vi "SetGreenLevel.vi"(0 "error in":errorcluster, 2 "Green Light \nLevel":sgl, 3 "node":string) -> (1 "error out":errorcluster)   [LabVIEW 2015]
doc: "Sets the green light on Baxter's head to a given level"
uses:
  ROS/Code/Console/Servers/ServerSubs/TopicDef.ctl
  ROS/Code/SubVIs/_ROSDirection.ctl
  ROS/MessageBuilding/std_msgs/subs/float32Scalar.vi
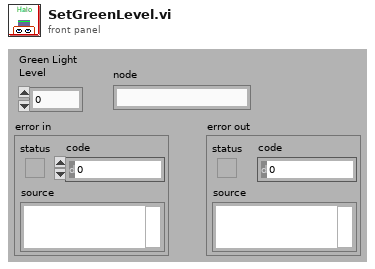
[diagram p1: front panel]
types:
  T1 = typedef "TopicDef.ctl" = cluster{"Topic":string, "Type":string, "Action":T2, "Update (ms)":u16, "queue size":u16}
  T2 = typedef "_ROSDirection.ctl" = enum16{"Node", "Publisher", "Subscriber", "ServiceClient", "ServiceProvider"}
  T3 = typedef "_ROSControl.ctl" = cluster{"topic port":u16, "Node":string, "topic":string, "type":string, "node port":u16, "error ":errorcluster, "Direction":T2, "Update (ms)":u16, "FIFO size":u16}
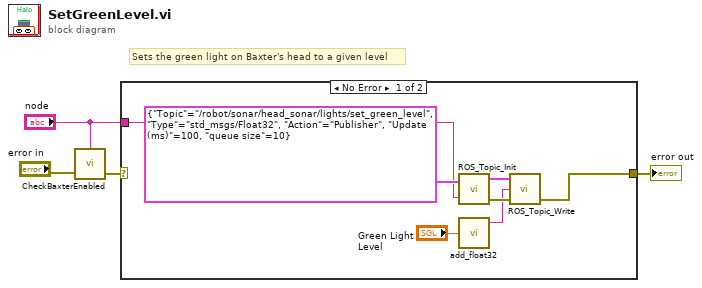
[diagram p0: block diagram]
diagram:
  # "Sets the green light on Baxter's head to a given level"
  n1 = call "CheckBaxterEnabled.vi"("error in"="error in", "node"="node") -> ("error out"=w2:errorcluster)  [unwired: 2 in]
  n2 = case shown="No Error" w2 {
    selector: w2 -> [_ w12]
    tunnel: [w5 w12] -> w4
    tunnel: "node" -> [w8 _]
    frame No Error {
      n3 = call "ROS_Topic_Init.vi"("Definitions"=T1 {"Topic"="/robot/sonar/head_sonar/lights/set_green_level", "Type"="std_msgs/Float32", "Action"=enum."Publisher", "Update (ms)"=100, "queue size"=10}, "node"=w8) -> ("ROS out"=w11:T3, "error out"=w7:errorcluster)  [unwired: 1 in]
      n4 = call-poly "add_float32.vi"("Numeric"="Green Light \nLevel") -> ("msg out"=w6:string)  [unwired: 4 in]
      n5 = call "ROS_Topic_Write.vi"("error in (no error)"=w7, "Msg in"=w6, "ROS in"=w11) -> ("error out"=w5:errorcluster)  [unwired: 1 in, 1 out]
    }
    frame Error {
    }
  }
  "error out" <- w4
